vi "UHR-Fleezers Control (host) - 12.6.vi"() -> ()   [LabVIEW 2012] (continued)
        n1396 = property on="Green Laser ON" class="Bool (strict)"("Val(Sgnl)"="Green Laser ON/OFF") -> ()  [unwired: 2 in, 2 out]
      }
      event "Laser interlacing mode", "Green Laser ON", "Red Laser ON", "Blue Laser ON": Value Change {
        n1397 = event-data() -> ()  [unwired: 7 out]
        n1398 = local write "Green Laser ON/OFF"("Green Laser ON") -> ()
        n1399 = local write "Blue Laser ON/OFF"("Blue Laser ON") -> ()
        n1400 = local write "Red Laser ON/OFF"("Red Laser ON") -> ()
        n1401 = case shown="True" "Green Laser ON" {
          tunnel: "Laser interlacing mode" -> [_ w2024]
          tunnel: [enum32{"Laser ON", "Laser OFF", "Interlace"}."Laser OFF" ("Green laser mode") w2024] -> w2000
          tunnel: [FALSE w2020] -> w1999
          frame False {
          }
          frame True {
            n1402 = local read "Green FB On/Off"() -> (w2021:bool)
            n1403 = Equal?(x=w2024, y=enum32{"Laser ON", "Laser OFF", "Interlace"}."Interlace") -> (x = y?=w2022:bool)
            n1404 = And(x=w2022, y=w2021) -> (x .and. y?=w2020:bool)
          }
        }
        n1405 = case shown="True" "Red Laser ON" {
          tunnel: "Laser interlacing mode" -> [_ w2017]
          tunnel: [enum32{"Laser ON", "Laser OFF", "Interlace"}."Laser OFF" ("Green laser mode") w2017] -> w1996
          tunnel: [FALSE w2013] -> w1995
          frame False {
          }
          frame True {
            n1406 = local read "Red FB On/Off"() -> (w2014:bool)
            n1407 = Equal?(x=w2017, y=enum32{"Laser ON", "Laser OFF", "Interlace"}."Interlace") -> (x = y?=w2015:bool)
            n1408 = And(x=w2015, y=w2014) -> (x .and. y?=w2013:bool)
          }
        }
        n1409 = case shown="True" "Blue Laser ON" {
          tunnel: "Laser interlacing mode" -> [_ w2008]
          tunnel: [enum32{"Laser ON", "Laser OFF", "Interlace"}."Laser OFF" ("Green laser mode") w2008] -> w1992
          tunnel: [FALSE w2006] -> w1991
          frame False {
          }
          frame True {
            n1410 = local read "Blue FB On/Off"() -> (w2007:bool)
            n1411 = Equal?(x=w2008, y=enum32{"Laser ON", "Laser OFF", "Interlace"}."Interlace") -> (x = y?=w2009:bool)
            n1412 = And(x=w2009, y=w2007) -> (x .and. y?=w2006:bool)
          }
        }
        n1413 = xnode "Read/Write Control"("FPGA VI Reference In"=w2003, "error in"=w2001, "Operating Mode"=w2000, "Operating Mode 2"=w2000, "Green FB On/Off"=w1999, "Red Laser Operating Mode"=w1996, "RI Operating Mode 2"=w1996, "Red FB On/Off"=w1995, "BI Operating Mode (AO)"=w1992, "Blue Laser Operating Mode (D)"=w1992, "Blue FB On/Off"=w1991) -> ("error out"=w2002:errorcluster)  [unwired: 1 out]
      }
      event "Invert laser interlacing": Value Change {
        n1414 = event-data() -> ()  [unwired: 7 out]
        n1415 = xnode "Read/Write Control"("FPGA VI Reference In"=w2028, "error in"=w2026, "Invert GI"="Invert laser interlacing", "Invert GI 2"="Invert laser interlacing", "Invert RI"="Invert laser interlacing", "Invert RI 2"="Invert laser interlacing", "Invert BI (AO)"="Invert laser interlacing", "Invert BI (D)"="Invert laser interlacing") -> ("error out"=w2027:errorcluster)  [unwired: 1 out]
      }
      event "Green FB Setpoint (mV)", "Green FB Gains", "Green FB On/Off", "Green Intensity % (FB OFF)", "Green int current ON count adj": Value Change {
        n1416 = event-data() -> ()  [unwired: 7 out]
        n1417 = local read "Green FB Setpoint (mV)"() -> (w2039:dbl)
        n1418 = Multiply(x=w2039, y=3.2767) -> (x*y=w2038:dbl)
        n1419 = local read "Green Intensity % (FB OFF)"() -> (w2042:dbl)
        n1420 = Multiply(x=w2042, y=655.35) -> (x*y=w2043:dbl)
        n1421 = To Unsigned Word Integer(number=w2043) -> (unsigned 16bit integer=w2041:u16)
        n1422 = local read "Green int current ON count adj"() -> (w2045:u32)
        n1423 = local read "Laser interlacing mode"() -> (w2035:enum32{"Laser ON", "Laser OFF", "Interlace"})
        n1424 = local read "Green FB Gains"() -> (w2032:T9)
        n1425 = local read "Green Laser ON"() -> (w2036:bool)
        n1426 = local read "Green FB On/Off"() -> (w2046:bool)
        n1427 = Equal?(x=w2035, y=enum32{"Laser ON", "Laser OFF", "Interlace"}."Interlace") -> (x = y?=w2033:bool)
        n1428 = Unbundle By Name(w2032) -> ("proportional gain (Kc)"=w2031:i16, "integral gain (Kc*Ts/Ti)"=w2030:i16, "derivative gain (Kc*Td/Ts)"=w2029:i16)
        n1429 = Compound Arithmetic op=AND(w2033, w2046, w2036) -> (w2037:bool)
        n1430 = xnode "Read/Write Control"("FPGA VI Reference In"=w2049, "error in"=w2048, "Green FB Setpoint"=w2038, "Green FB On/Off"=w2037, "Current Out"=w2041, "Green int current ON count adj"=w2045, "P3"=w2031, "I3"=w2030, "D3"=w2029) -> ("error out"=w2047:errorcluster)  [unwired: 1 out]
      }
      event "Blue FB Setpoint (mV)", "Blue FB Gains", "Blue FB On/Off", "Blue Intensity % (FB OFF)", "Blue int AO ON count adjust": Value Change {
        # "16 bit analog out"
        n1431 = event-data() -> ()  [unwired: 7 out]
        n1432 = Multiply(x="Blue FB Setpoint (mV)", y=3.2767) -> (x*y=w2063:dbl)
        n1433 = Multiply(x="Blue Intensity % (FB OFF)", y=655.35) -> (x*y=w2066:dbl)
        n1434 = To Unsigned Word Integer(number=w2066) -> (unsigned 16bit integer=w2065:u16)
        n1435 = local read "Laser interlacing mode"() -> (w2061:enum32{"Laser ON", "Laser OFF", "Interlace"})
        n1436 = Unbundle By Name("Blue FB Gains") -> ("proportional gain (Kc)"=w2058:i16, "integral gain (Kc*Ts/Ti)"=w2057:i16, "derivative gain (Kc*Td/Ts)"=w2056:i16)
        n1437 = local read "Blue Laser ON"() -> (w2050:bool)
        n1438 = Equal?(x=w2061, y=enum32{"Laser ON", "Laser OFF", "Interlace"}."Interlace") -> (x = y?=w2059:bool)
        n1439 = Compound Arithmetic op=AND(w2059, "Blue FB On/Off", w2050) -> (w2062:bool)
        n1440 = xnode "Read/Write Control"("FPGA VI Reference In"=w2070, "error in"=w2069, "Blue FB Setpoint"=w2063, "Blue FB On/Off"=w2062, "BI Current Out"=w2065, "Blue current ON count adj (AO)"="Blue int AO ON count adjust", "P5"=w2058, "I5"=w2057, "D5"=w2056) -> ("error out"=w2068:errorcluster)  [unwired: 1 out]
      }
      event "Red FB Setpoint (mV)", "Red FB Gains", "Red FB On/Off", "Red Intensity % (FB OFF)": Value Change {
        n1441 = event-data() -> ()  [unwired: 7 out]
        n1442 = local read "Red FB Setpoint (mV)"() -> (w2082:dbl)
        n1443 = Multiply(x=w2082, y=3.2767) -> (x*y=w2081:dbl)
        n1444 = local read "Red Intensity % (FB OFF)"() -> (w2071:dbl)
        n1445 = Multiply(x=w2071, y=655.35) -> (x*y=w2085:dbl)
        n1446 = To Unsigned Word Integer(number=w2085) -> (unsigned 16bit integer=w2084:u16)
        n1447 = local read "Laser interlacing mode"() -> (w2078:enum32{"Laser ON", "Laser OFF", "Interlace"})
        n1448 = local read "Red FB Gains"() -> (w2075:T9)
        n1449 = local read "Red Laser ON"() -> (w2079:bool)
        n1450 = local read "Red FB On/Off"() -> (w2087:bool)
        n1451 = Equal?(x=w2078, y=enum32{"Laser ON", "Laser OFF", "Interlace"}."Interlace") -> (x = y?=w2076:bool)
        n1452 = Unbundle By Name(w2075) -> ("proportional gain (Kc)"=w2074:i16, "integral gain (Kc*Ts/Ti)"=w2073:i16, "derivative gain (Kc*Td/Ts)"=w2072:i16)
        n1453 = Compound Arithmetic op=AND(w2076, w2087, w2079) -> (w2080:bool)
        n1454 = xnode "Read/Write Control"("FPGA VI Reference In"=w2090, "error in"=w2089, "Red FB Setpoint"=w2081, "Red FB On/Off"=w2080, "RI Current Out"=w2084, "P4"=w2074, "I4"=w2073, "D4"=w2072) -> ("error out"=w2088:errorcluster)  [unwired: 1 out]
      }
      event "+ phase (APD 1 Gate)", "- phase (APD 1 Gate)", "+ phase (APD 2 Gate)", "- phase (APD 2 Gate)", "+ phase (APD 3 Gate)", "- phase (APD 3 Gate)", "+ phase (APD Acq)", "- phase (APD Acq)": Value Change {
        n1455 = event-data() -> ()  [unwired: 7 out]
        n1456 = local read "Phase Adj. (APD 1 Gate)"() -> (w2110:i16)
        n1457 = Or(x="- phase (APD 1 Gate)", y="+ phase (APD 1 Gate)") -> (x .or. y?=w2112:bool)
        n1458 = Negate(x=w2110) -> (-x=w2117:i16)
        n1459 = Select(t=w2117, s="+ phase (APD 1 Gate)", f=w2110) -> (s? t:f=w2116:i16)
        n1460 = local read "Phase Adj. (APD 2 Gate)"() -> (w2107:i16)
        n1461 = Or(x="- phase (APD 2 Gate)", y="+ phase (APD 2 Gate)") -> (x .or. y?=w2105:bool)
        n1462 = Negate(x=w2107) -> (-x=w2109:i16)
        n1463 = Select(t=w2109, s="+ phase (APD 2 Gate)", f=w2107) -> (s? t:f=w2106:i16)
        n1464 = Negate(x="Phase Adj. (APD 3 Gate)") -> (-x=w2104:i16)
        n1465 = Or(x="- phase (APD 3 Gate)", y="+ phase (APD 3 Gate)") -> (x .or. y?=w2100:bool)
        n1466 = Select(t=w2104, s="+ phase (APD 3 Gate)", f="Phase Adj. (APD 3 Gate)") -> (s? t:f=w2101:i16)
        n1467 = local read "Phase Adj. (APD Acq)"() -> (w2098:i16)
        n1468 = Or(x="- phase (APD Acq)", y="+ phase (APD Acq)") -> (x .or. y?=w2096:bool)
        n1469 = Negate(x=w2098) -> (-x=w2099:i16)
        n1470 = Select(t=w2099, s="+ phase (APD Acq)", f=w2098) -> (s? t:f=w2097:i16)
        n1471 = xnode "Read/Write Control"("FPGA VI Reference In"=w2119, "error in"=w2118, "Phase count adjustment (APD 1 Gate)"=w2116, "Phase count adjustment (APD 2 Gate)"=w2106, "Phase count adjustment (APD 3 Gate)"=w2101, "Phase Count Adjustment (APD Acq)"=w2097) -> ("FPGA VI Reference Out"=w2114:T20, "error out"=w2115:errorcluster)
        n1472 = xnode "Read/Write Control"("FPGA VI Reference In"=w2114, "error in"=w2115, "+ phase (APD 1 Gate)"=w2112, "+ phase (APD 2 Gate)"=w2105, "+ phase (APD 3 Gate)"=w2100, "+ phase (APD Acq)"=w2096) -> ("error out"=w2113:errorcluster)  [unwired: 1 out]
      }
      event "Invert APD Gate", "APD Gate ON Count", "APD Gate OFF Count", "APD Gate", "APD Integration Time (s)", "APD AO Scale Factor", "Duty Frequency (ON 1/N cycles)", "Interlace ON count", "Interlace OFF count": Value Change {
        n1473 = event-data() -> ()  [unwired: 7 out]
        n1474 = Add(x="Interlace ON count", y="Interlace OFF count") -> (x+y=w2125:u16)
        n1475 = Add(x="APD Gate ON Count", y="APD Gate OFF Count") -> (x+y=w2136:u16)
        n1476 = Multiply(x="Duty Frequency (ON 1/N cycles)", y=w2125) -> (x*y=w2121:u16)
        "Green AI Count" <- w2121
        "Red AI Count" <- w2121
        "Blue AI Count" <- w2121
        n1477 = Subtract(x=w2121, y="Interlace ON count") -> (x-y=w2124:u16)
        n1478 = Multiply(x=w2136, y="Duty Frequency (ON 1/N cycles)") -> (x*y=w2135:u16)
        n1479 = Subtract(x=w2135, y="APD Gate ON Count") -> (x-y=w2134:u16)
        n1480 = local read "DMA Update Period (s)"() -> (w2137:dbl)
        n1481 = Multiply(x="APD Integration Time (s)", y=40000000.0) -> (x*y=w2141:dbl)
        n1482 = Reciprocal(x="APD Integration Time (s)") -> (1/x=→"APD Acq Rate (Hz)":dbl)
        n1483 = To Unsigned Long Integer(number=w2141) -> (unsigned 32bit integer=w2127:u32)
        "APD Int. Count" <- w2127
        n1484 = local read "Number of APDs"() -> (w2120:u8)
        n1485 = Divide(x=w2137, y="APD Integration Time (s)") -> (x/y=w2139:dbl)
        n1486 = Multiply(x=w2120, y=w2139) -> (x*y=w2138:dbl)
        n1487 = local write "APD Samples/FIFO Acq."(w2139) -> ()
        n1488 = local write "APD Elements/DMA read"(w2138) -> ()
        n1489 = xnode "Read/Write Control"("FPGA VI Reference In"=w2145, "error in"=w2144, "Invert APD Gate"="Invert APD Gate", "APD Gate ON Count"="APD Gate ON Count", "APD Gate OFF Count"=w2134, "APD Acq Rate Count"=w2127, "APD Gate Operating Mode"="APD Gate", "APD AO scale factor"="APD AO Scale Factor", "Green interlace ON count"="Interlace ON count", "Green interlace OFF count"=w2124, "Green interlace ON count 2"="Interlace ON count", "Green interlace OFF count 2"=w2124, "Green FB Count"=w2121, "Red interlace ON count"="Interlace ON count", "Red interlace OFF count"="Interlace OFF count", "Blue ON count (AO)"="Interlace ON count", "Blue OFF count (AO)"="Interlace OFF count", "Blue interlace OFF count (D)"="Interlace OFF count", "Blue interlace ON count (D)"="Interlace ON count") -> ("error out"=w2143:errorcluster)  [unwired: 1 out]
      }
      event "Neg. TTrig FPGA": Value Change {
        n1490 = event-data() -> ()  [unwired: 7 out]
        n1491 = xnode "Read/Write Control"("FPGA VI Reference In"=w2148, "error in"=w2147, "TTrig Negate Pos"="Neg. TTrig FPGA") -> ()  [unwired: 2 out]
      }
      event "Test ttrig": Value Change {
        n1492 = event-data() -> ()  [unwired: 7 out]
        n1493 = xnode "Read/Write Control"("FPGA VI Reference In"=w2152, "error in"=w2151, "TTrig?"=TRUE) -> ("error out"=w2150:errorcluster)  [unwired: 1 out]
      }
      event "Number of F/B Scans (AOD)", "Scan Speed (nm/s)", "Scan BD", "Initial delta (MHz)", "Step Size (nm)", "Scan Range (nm)": Value Change {
        w2215 = 123.0  # AOM cal (nm/MHz)
        n1494 = event-data() -> ()  [unwired: 7 out]
        n1495 = local read "BD 1 Frequency 1 (MHz)"() -> (w2198:dbl)
        n1496 = local read "AOM X Cal (nm/MHz)"() -> (w2190:dbl)
        n1497 = local read "X RF Frequency Limits (MHz)"() -> (w2202:T16)
        n1498 = local read "Y RF Frequency Limits (MHz)"() -> (w2199:T16)
        n1499 = local read "BD 2 Frequency 1 (MHz)"() -> (w2204:dbl)
        n1500 = Negate(x="Scan Range (nm)") -> (-x=w2168:dbl)
        n1501 = Divide(x=w2168, y=w2190) -> (x/y=w2172:dbl)
        n1502 = Select(t=w2202, s="Scan BD", f=w2199) -> (s? t:f=w2201:T16)
        n1503 = Select(t=w2198, s="Scan BD", f=w2204) -> (s? t:f=w2203:dbl)
        n1504 = Unbundle By Name(w2201) -> ("Maximum"=w2210:dbl, "Minimum"=w2209:dbl)
        n1505 = Add(x=w2172, y=w2203) -> (x+y=w2207:dbl)
        n1506 = Divide(x=w2168, y="Step Size (nm)") -> (x/y=w2187:dbl)
        n1507 = Divide(x="Step Size (nm)", y=w2190) -> (x/y=w2196:dbl)
        n1508 = Absolute Value(x=w2187) -> (abs(x)=w2171:dbl)
        n1509 = Sign(1:w2168) -> (0:w2169:dbl)
        n1510 = In Range and Coerce(upper limit=w2210, x=w2207, lower limit=w2209) -> (coerced(x)=w2206:dbl, In Range?=w2208:bool)
        n1511 = To Unsigned Quad Integer(1:w2171) -> (0:w2186:u64)
        "Scan steps (AOD)" <- w2186
        n1512 = call "IR AOM freq to word.vi"("Frequency In (MHz)"=w2196) -> ("Frequency Word Out (double)"=w2193:dbl)
        n1513 = Multiply(x=w2169, y=w2193) -> (x*y=w2170:dbl)
        n1514 = Subtract(x=w2207, y=w2206) -> (x-y=w2205:dbl)
        n1515 = To Quad Integer(1:w2170) -> (0:w2192:i64)
        "Incr. int (AOD)" <- w2192
        n1516 = Subtract(x=w2172, y=w2205) -> (x-y=w2191:dbl)
        "Scan Range (MHz)" <- w2191
        n1517 = Select(t=w2172, s=w2208, f=w2191) -> (s? t:f=w2211:dbl)
        n1518 = Multiply(x=w2191, y=w2190) -> (x*y=w2189:dbl)
        n1519 = Decrement(x=w2186) -> (x-1=w2239:u64)
        n1520 = Negate(x=w2189) -> (-x=w2185:dbl)
        n1521 = local write "Scan Range (nm)"(w2185) -> ()
        n1522 = Divide(x=w2211, y=w2239) -> (x/y=w2195:dbl)
        "Scan Increment (MHz)" <- w2195
        n1523 = call "IR AOM freq to word.vi"("Frequency In (MHz)"=w2195) -> ("Frequency Word Out (double)"=w2194:dbl)
        n1524 = Divide(x="Step Size (nm)", y="Scan Speed (nm/s)") -> (x/y=w2182:dbl)
        n1525 = To Quad Integer(1:w2194) -> ()  [unwired: 1 out]
        n1526 = local read "Number Interlace Sets"() -> (w2166:u8)
        n1527 = local read "AI Count (ticks)"() -> (w2167:u16)
        n1528 = local read "Total Counts (ticks)"() -> (w2165:u16)
        n1529 = local read "# Samples/trap"() -> (w2197:u32)
        n1530 = Multiply(x=w2167, y=w2166) -> (x*y=w2164:u16)
        n1531 = Divide(x=w2165, y=w2164) -> (x/y=w2163:dbl)
        n1532 = Select(t=w2198, s="Scan BD", f=w2204) -> (s? t:f=w2236:dbl)
        "Initial freq. (MHz)" <- w2236
        n1533 = Add(x=w2211, y=w2236) -> (x+y=→"Final freq. (MHz)":dbl)
        n1534 = Divide(x=w2165, y=40000000.0) -> (x/y=w2181:dbl)
        n1535 = Divide(x=w2182, y=w2181) -> (x/y=w2180:dbl)
        n1536 = To Unsigned Quad Integer(1:w2180) -> (0:w2155:u64)
        n1537 = Quotient & Remainder(x=w2155, y=u64 2) -> (x-y*floor(x/y)=w2159:u64)  [unwired: 1 out]
        n1538 = Equal?(x=w2159, y=u64 0) -> (x = y?=w2157:bool)
        n1539 = Decrement(x=w2155) -> (x-1=w2156:u64)
        n1540 = Select(t=w2155, s=w2157, f=w2156) -> (s? t:f=w2154:u64)
        "Cycles/step (AOD)" <- w2154
        n1541 = xnode "Read/Write Control"("FPGA VI Reference In"=w2247, "error in"=w2246, "Scan steps"=w2186, "Number of scans"="Number of F/B Scans (AOD)", "Cycles per step"=w2154, "Scan freq.  increment"=w2192, "Scan BD"="Scan BD") -> ("error out"=w2245:errorcluster)  [unwired: 1 out]
        n1542 = Multiply(x=w2186, y=w2154) -> (x*y=w2240:u64)
        n1543 = Multiply(x=w2240, y=u64 2) -> (x*y=w2162:u64)
        n1544 = Multiply(x=w2163, y=w2162) -> (x*y=w2161:dbl)
        "Data points/scan (f/b)" <- w2161
        n1545 = Multiply(x=w2161, y="Number of F/B Scans (AOD)") -> (x*y=w2243:dbl)
        "Data points/scans" <- w2243
        n1546 = Divide(x=w2243, y=w2197) -> (x/y=→"N sets should be saved":dbl)
        n1547 = Multiply(x=w2240, y=w2181) -> (x*y=w2179:dbl)
        "Time/Scan (s) (AOD)" <- w2179
        n1548 = Select(t=w2211, s="Scan BD", f=0.0) -> (s? t:f=w2237:dbl)
        n1549 = Select(t=0.0, s="Scan BD", f=w2211) -> (s? t:f=w2233:dbl)
        n1550 = local read "BD 2 Frequency 2 (MHz)"() -> (w2229:dbl)
        n1551 = local read "BD 1 Frequency 2 (MHz)"() -> (w2232:dbl)
        n1552 = Add(x=w2233, y=w2204) -> (x+y=w2230:dbl)
        n1553 = Add(x=w2198, y=w2237) -> (x+y=w2231:dbl)
        n1554 = Multiply(x=w2179, y=2.0) -> (x*y=w2178:dbl)
        n1555 = Multiply(x=w2178, y="Number of F/B Scans (AOD)") -> (x*y=w2175:dbl)
        n1556 = Divide(x=w2175, y=60.0) -> (x/y=→"Time to Finish All (min)":dbl)
        n1557 = Add(x="Trap 2 Bead Size (nm)", y="Trap 1 Bead Size (nm)") -> (x+y=w2219:dbl)
        n1558 = Divide(x=w2219, y=2.0) -> (x/y=w2213:dbl)
        n1559 = local read "Initial delta (MHz)"() -> (w2216:dbl)
        n1560 = Subtract(x=w2230, y=w2229) -> (x-y=w2227:dbl)
        n1561 = Subtract(x=w2231, y=w2232) -> (x-y=w2228:dbl)
        n1562 = Square(x=w2227) -> (x^2=w2226:dbl)
        n1563 = Square(x=w2228) -> (x^2=w2225:dbl)
        n1564 = Add(x=w2225, y=w2226) -> (x+y=w2224:dbl)
        n1565 = Square Root(x=w2224) -> (sqrt(x)=w2223:dbl)
        "Final delta (MHz)" <- w2223
        n1566 = Multiply(x=w2215, y=w2223) -> (x*y=w2222:dbl)
        n1567 = Multiply(x=w2216, y=w2215) -> (x*y=w2214:dbl)
        n1568 = Subtract(x=w2214, y=w2213) -> (x-y=→"Initial sep (nm)":dbl)
        n1569 = Subtract(x=w2222, y=w2213) -> (x-y=→"Final sep (nm)":dbl)
      }
      event "Freq or Amp switch first", "Swap F1 and F2", "Freq switch delay", "Amp switch delay": Value Change {
        n1570 = event-data() -> ()  [unwired: 7 out]
        n1571 = local read "Amp switch delay"() -> (w2248:u16)
        n1572 = local read "Swap F1 and F2"() -> (w2249:bool)
        n1573 = xnode "Read/Write Control"("FPGA VI Reference In"=w2252, "error in"=w2251, "Swap F1 and F2"=w2249, "Amp switch delay"=w2248) -> ("error out"=w2250:errorcluster)  [unwired: 1 out]
      }
      event "Scan steps (MCL)", "Number of scans (MCL)", "Scan Range (V)\n(of steps)", "2D or 1D Scan", "N APD Samp/step", "Fast Scan Dir", "Continuous MCL Scanning", "Scan lines (y)": Value Change {
        w2254 = 32767.0 ("y")
        n1574 = event-data() -> ()  [unwired: 7 out]
        n1575 = Select(t="Scan lines (y)", s="2D or 1D Scan", f="Number of scans (MCL)") -> (s? t:f=w2259:u64)
        n1576 = Decrement(x="Scan steps (MCL)") -> (x-1=w2275:u64)
        n1577 = Divide(x="Scan Range (V)\n(of steps)", y=w2275) -> (x/y=w2274:dbl)
        "Desired Scan Incr (V)" <- w2274
        n1578 = local read "APD Integration Time (s)"() -> (w2267:dbl)
        n1579 = Multiply(x=w2274, y=w2254) -> (x*y=w2283:dbl)
        n1580 = Divide(x=w2283, y=10.0) -> (x/y=w2273:dbl)
        "Desired incr (int)" <- w2273
        n1581 = local read "Update Count (MCL)"() -> (w2279:u32)
        n1582 = Round Toward -Infinity(1:w2273) -> (0:w2282:dbl)
        n1583 = To Word Integer(number=w2282) -> (16bit integer=w2257:i16)
        "Actual Incr. int (MCL)" <- w2257
        n1584 = Multiply(x=w2267, y=40000000.0) -> (x*y=w2280:dbl)
        n1585 = Divide(x=w2280, y=w2279) -> (x/y=w2278:dbl)
        n1586 = Multiply(x=i16 10, y=w2257) -> (x*y=w2255:i16)
        n1587 = Multiply(x="N APD Samp/step", y=w2278) -> (x*y=w2277:dbl)
        "Cycles/step (MCL)" <- w2277
        n1588 = Divide(x=w2255, y=w2254) -> (x/y=→"Actual MCL Inc (V)":dbl)
        n1589 = Multiply(x="N APD Samp/step", y="Scan steps (MCL)") -> (x*y=w2269:dbl)
        n1590 = local read "APD Samples/FIFO Acq."() -> (w2266:dbl)
        n1591 = Multiply(x=w2269, y=u64 2) -> (x*y=w2268:dbl)
        "Data points/scan (f+b)" <- w2268
        n1592 = Multiply(x=w2268, y=w2259) -> (x*y=w2286:dbl)
        "Data points/scans (MCL)" <- w2286
        n1593 = Multiply(x=w2267, y=w2268) -> (x*y=w2260:dbl)
        "Time/f+b scan (s) (MCL)" <- w2260
        n1594 = Divide(x=w2286, y=w2266) -> (x/y=→"N sets should be saved (MCL)":dbl)
        n1595 = Multiply(x=w2260, y=w2259) -> (x*y=→"Total Time (s)":dbl)
        n1596 = Not(x="Fast Scan Dir") -> (.not. x?=w2264:bool)
        n1597 = xnode "Read/Write Control"("FPGA VI Reference In"=w2290, "error in"=w2289, "Scan steps (MCL)"="Scan steps (MCL)", "Number of scans (MCL)"=w2259, "Cycles per step (MCL)"=w2277, "Scan freq.  increment (MCL)"=w2257, "1D or 2D Scan?"="2D or 1D Scan", "MCL Scan Axis"=w2264, "Cont. Scan (MCL)"="Continuous MCL Scanning") -> ("error out"=w2288:errorcluster)  [unwired: 1 out]
      }
      event "Read Cal": Value Change {
        w2292 = 1000.0 ("y")
        n1598 = event-data() -> ()  [unwired: 7 out]
        n1599 = local read "Save file name"() -> (w2317:path)
        n1600 = local write "Read Cal"(FALSE ("Read Cal")) -> ()
        n1601 = Strip Path(path=w2317) -> (stripped path=w2316:path)  [unwired: 1 out]
        n1602 = Path To String(path=w2316) -> (string=w2315:string)
        n1603 = Concatenate Strings(w2315, "\\current.cal" ("string")) -> (w2313:string)
        n1604 = String To Path(string=w2313) -> (path=w2312:path)
        n1605 = Open/Create/Replace File(file path (use dialog)=w2312, operation (0:open)=T29."open", access (0:read/write)=enum16{"read/write", "read-only", "write-only"}."read-only") -> (refnum out=w2320:refnum<file>, error out=w2306:errorcluster)  [unwired: 1 in, 3 out]
        n1606 = Deny Access(4:w2306, 7:w2320) -> (0:w2305:errorcluster, 3:w2311:refnum<file>)  [unwired: 1 out]
        n1607 = Read from Binary File(5:0.0, 8:w2305, 9:T28."big-endian, network order" ("byte order (0:big-endian, network order)"), 10:-1 ("count (1)"), 11:w2311) -> (0:w2304:errorcluster, 2:w2302:dbl[], 3:w2307:refnum<file>)  [unwired: 2 out]
        n1608 = Array To Cluster(array=w2302) -> (cluster=w2301:T31)
        n1609 = Unbundle(w2301) -> ("[0]"=w2300:dbl, "[1]"=w2299:dbl, "[2]"=w2298:dbl, "[3]"=w2297:dbl, "[4]"=w2296:dbl, "[5]"=w2295:dbl)
        n1610 = Close File(refnum=w2307, error in=w2304) -> (error out=→"Read cal error":errorcluster)  [unwired: 1 out]
        n1611 = Multiply(x=w2295, y=w2292) -> (x*y=w2293:dbl)
        n1612 = local write "T2 kappa_x (pN/nm)"(w2297) -> ()
        n1613 = local write "T1 kappa_x (pN/nm)"(w2298) -> ()
        n1614 = local write "T1 alpha_x (nm/V)"(w2300) -> ()
        n1615 = local write "T2 alpha_x (nm/V)"(w2299) -> ()
        n1616 = Multiply(x=w2296, y=w2292) -> (x*y=w2294:dbl)
        n1617 = local write "T1 offset_x (mV)"(w2294) -> ()
        n1618 = local write "T2 offset_x (mV)"(w2293) -> ()
      }
      event "Abort MCL Scan": Value Change {
        n1619 = event-data() -> ()  [unwired: 7 out]
        n1620 = local write "MCL Scanning"(FALSE ("MCL Scanning")) -> ()
        n1621 = xnode "Read/Write Control"("FPGA VI Reference In"=w2325, "error in"=w2324, "Abort scan (MCL)"="Abort MCL Scan") -> ("error out"=w2323:errorcluster)  [unwired: 1 out]
      }
      event "Update Count (MCL)": Value Change {
        n1622 = event-data() -> ()  [unwired: 7 out]
        n1623 = xnode "Read/Write Control"("FPGA VI Reference In"=w2329, "error in"=w2328, "MCL count"="Update Count (MCL)") -> ("error out"=w2327:errorcluster)  [unwired: 1 out]
      }
      event "+ phase (MCL)", "- phase (MCL)": Value Change {
        n1624 = event-data() -> ()  [unwired: 7 out]
        n1625 = Or(x="- phase (MCL)", y="+ phase (MCL)") -> (x .or. y?=w2332:bool)
        n1626 = Negate(x="Phase adjust (MCL)") -> (-x=w2338:i16)
        n1627 = Select(t=w2338, s="+ phase (MCL)", f="Phase adjust (MCL)") -> (s? t:f=w2336:i16)
        n1628 = xnode "Read/Write Control"("FPGA VI Reference In"=w2340, "error in"=w2339, "Phase count adjustment (MCL)"=w2336) -> ("FPGA VI Reference Out"=w2333:T20, "error out"=w2334:errorcluster)
        n1629 = xnode "Read/Write Control"("FPGA VI Reference In"=w2333, "error in"=w2334, "+ phase (MCL)"=w2332) -> ("error out"=w2331:errorcluster)  [unwired: 1 out]
      }
      event "Abort AOD Scan": Value Change {
        n1630 = event-data() -> ()  [unwired: 7 out]
        n1631 = xnode "Read/Write Control"("FPGA VI Reference In"=w2344, "error in"=w2343, "Abort scan"="Abort AOD Scan") -> ("error out"=w2342:errorcluster)  [unwired: 1 out]
      }
      event "Continuous AOD Scanning": Value Change {
        n1632 = event-data() -> ()  [unwired: 7 out]
        n1633 = xnode "Read/Write Control"("FPGA VI Reference In"=w2348, "error in"=w2347, "Cont. Scan"="Continuous AOD Scanning") -> ("error out"=w2346:errorcluster)  [unwired: 1 out]
      }
      event "Index": Value Change {
        n1634 = event-data() -> ()  [unwired: 7 out]
        n1635 = call "Create new save file.vi"("Insert"="", "Ext"=".dat" ("string"), "Index In"="Index") -> ("Path Out"=→"Save file name":path, "Index Out"=w2349:dbl)
        "Save index" <- w2349
        n1636 = local write "Index"(w2349) -> ()
      }
      event "AO1", "AO2": Value Change {
        w2364 = 10.0 ("y")
        w2363 = 32767.0 ("y")
        n1637 = event-data() -> ()  [unwired: 7 out]
        n1638 = local read "AO2"() -> (w2362:dbl)
        n1639 = local read "AO1"() -> (w2359:dbl)
        n1640 = Multiply(x=w2359, y=w2363) -> (x*y=w2358:dbl)
        n1641 = Multiply(x=w2362, y=w2363) -> (x*y=w2361:dbl)
        n1642 = Divide(x=w2358, y=w2364) -> (x/y=w2357:dbl)
        n1643 = Divide(x=w2361, y=w2364) -> (x/y=w2360:dbl)
        n1644 = To Word Integer(number=w2357) -> (16bit integer=w2365:i16)
        n1645 = To Word Integer(number=w2360) -> (16bit integer=w2366:i16)
        n1646 = xnode "Read/Write Control"("FPGA VI Reference In"=w2356, "error in"=w2355, "AO1"=w2365, "AO2"=w2366) -> ("error out"=w2354:errorcluster)  [unwired: 1 out]
      }
      event "Inject Pump 1": Value Change {
        n1647 = event-data() -> ()  [unwired: 7 out]
        n1648 = local read "Use Harvard pumps\nfor beads (else Chemyx)"() -> (w2368:bool)
        n1649 = case shown="True" w2368 {
          tunnel: "Inject Pump 1" -> [w2372 w2410]
          tunnel: w2367 -> [_ w2411]
          frame False {
            n1650 = local read "Pump write delay (ms)"() -> (w2371:dbl)
            n1651 = local read "Chemyx Syringe Pump Serial Port"() -> (w2370:refnum<visa-resource-name>)
            n1652 = case shown="True" w2372 {
              tunnel: w2371 -> [w2378 w2392]
              tunnel: w2370 -> [w2375 w2391]
              frame False {
                n1653 = flat-sequence {
                  tunnel: w2375 -> [w2379]
                  tunnel: [w2379] -> w2376
                  tunnel: w2378 -> [_]
                  tunnel: [w2382] -> w2377
                  tunnel: w2376 -> [w2382]
                  tunnel: w2377 -> [w2383]
                  tunnel: [w2383] -> w2373
                  tunnel: [w2385] -> w2374
                  tunnel: w2373 -> [w2385]
                  tunnel: w2374 -> [w2387]
                  frame #0 {
                    n1654 = call "Write to pump.vi"("string"="enter pump1", "VISA resource name"=w2379) -> ()  [unwired: 1 out]
                  }
                  frame #1 {
                    n1655 = Wait (ms)(milliseconds to wait="Pump pause delay (ms)") -> ()  [unwired: 1 out]
                  }
                  frame #2 {
                    n1656 = call "Write to pump.vi"("string"="stop", "VISA resource name"=w2383) -> ()  [unwired: 1 out]
                  }
                  frame #3 {
                    n1657 = Wait (ms)(milliseconds to wait=u32 500) -> ()  [unwired: 1 out]
                  }
                  frame #4 {
                    n1658 = call "Write to pump.vi"("string"="stop", "VISA resource name"=w2387) -> ()  [unwired: 1 out]
                  }
                }
              }
              frame True {
                n1659 = flat-sequence {
                  tunnel: w2391 -> [w2401]
                  tunnel: w2392 -> [w2396]
                  tunnel: w2392 -> [w2403]
                  tunnel: w2391 -> [w2404]
                  tunnel: [w2404] -> w2389
                  tunnel: [w2406] -> w2390
                  tunnel: w2389 -> [w2406]
                  tunnel: w2390 -> [w2408]
                  frame #0 {
                    n1660 = local read "All Pump Parameters"() -> (w2395:T5)
                    n1661 = Unbundle By Name(w2395) -> ("Pump 1"=w2402:T32)
                    n1662 = call "Set pump parameters.vi"("Pump write delay (ms)"=w2396, "Volume (uL)"="Ch 1 Inject Volume (uL)", "Rate (uL/h)"="Ch 1 Inject Rate (ul/h)", "Units"=4.0, "Pump #"=1.0, "Pump Parameters In"=w2402, "VISA resource name"=w2401) -> ("Pump Parameters Out"=w2394:T32)  [unwired: 3 in]
                    n1663 = Bundle By Name(cluster=w2395, "Pump 1"=w2394) -> (w2393:T5)
                    n1664 = local write "All Pump Parameters"(w2393) -> ()
                  }
                  frame #1 {
                    n1665 = Wait (ms)(milliseconds to wait=w2403) -> ()  [unwired: 1 out]
                  }
                  frame #2 {
                    n1666 = call "Write to pump.vi"("string"="start", "VISA resource name"=w2404) -> ()  [unwired: 1 out]
                  }
                  frame #3 {
                    n1667 = Wait (ms)(milliseconds to wait=u32 500) -> ()  [unwired: 1 out]
                  }
                  frame #4 {
                    n1668 = call "Write to pump.vi"("string"="start", "VISA resource name"=w2408) -> ()  [unwired: 1 out]
                  }
                }
              }
            }
          }
          frame True {
            n1669 = case shown="False" w2410 {
              tunnel: w2411 -> [w2412 w2422]
              frame False {
                n1670 = flat-sequence {
                  tunnel: w2412 -> [w2414]
                  frame #0 {
                    n1671 = local write "Flushing P1"(FALSE ("Flushing P1")) -> ()
                    n1672 = Concatenate Strings("stop" ("string"), "\r") -> (w2416:string)
                    n1673 = VISA Write(VISA resource name=w2414, write buffer=w2416) -> ()  [unwired: 1 in, 3 out]
                  }
                  frame #1 {
                    n1674 = property on="Clear Volume P1" class="Bool (strict)"("Val(Sgnl)"=TRUE ("Value (Signaling)")) -> ()  [unwired: 2 in, 2 out]
                  }
                }
              }
              frame True {
                n1675 = local read "Normal Flow Rate (ul/h) P1"() -> (w2420:dbl)
                n1676 = Number To Decimal String(number=w2420) -> (decimal integer string=w2426:string)  [unwired: 1 in]
                n1677 = Concatenate Strings("irate  " ("string"), w2426, " u/h" ("string"), "\r") -> (w2424:string)
                n1678 = VISA Write(VISA resource name=w2422, write buffer=w2424) -> (VISA resource name out=w2421:refnum<visa-resource-name>)  [unwired: 1 in, 2 out]
                n1679 = Concatenate Strings("irun" ("string"), "\r") -> (w2428:string)
                n1680 = VISA Write(VISA resource name=w2421, write buffer=w2428) -> ()  [unwired: 1 in, 3 out]
              }
            }
          }
        }
      }
      event "Inject Pump 3": Value Change {
        n1681 = event-data() -> ()  [unwired: 7 out]
        n1682 = local read "Use Harvard pumps\nfor beads (else Chemyx)"() -> (w2431:bool)
        n1683 = case shown="True" w2431 {
          tunnel: "Inject Pump 3" -> [w2435 w2474]
          tunnel: w2430 -> [_ w2473]
          frame False {
            n1684 = local read "Pump write delay (ms)"() -> (w2434:dbl)
            n1685 = case shown="True" w2435 {
              tunnel: w2434 -> [w2441 w2455]
              tunnel: "Chemyx Syringe Pump Serial Port" -> [w2438 w2454]
              frame False {
                n1686 = flat-sequence {
                  tunnel: w2438 -> [w2442]
                  tunnel: [w2442] -> w2439
                  tunnel: w2441 -> [_]
                  tunnel: [w2445] -> w2440
                  tunnel: w2439 -> [w2445]
                  tunnel: w2440 -> [w2446]
                  tunnel: [w2446] -> w2436
                  tunnel: [w2448] -> w2437
                  tunnel: w2436 -> [w2448]
                  tunnel: w2437 -> [w2450]
                  frame #0 {
                    n1687 = call "Write to pump.vi"("string"="enter pump3", "VISA resource name"=w2442) -> ()  [unwired: 1 out]
                  }
                  frame #1 {
                    n1688 = local read "Pump pause delay (ms)"() -> (w2444:u32)
                    n1689 = Wait (ms)(milliseconds to wait=w2444) -> ()  [unwired: 1 out]
                  }
                  frame #2 {
                    n1690 = call "Write to pump.vi"("string"="stop", "VISA resource name"=w2446) -> ()  [unwired: 1 out]
                  }
                  frame #3 {
                    n1691 = Wait (ms)(milliseconds to wait=u32 0) -> ()  [unwired: 1 out]
                  }
                  frame #4 {
                    n1692 = call "Write to pump.vi"("string"="stop", "VISA resource name"=w2450) -> ()  [unwired: 1 out]
                  }
                }
              }
              frame True {
                n1693 = flat-sequence {
                  tunnel: w2454 -> [w2464]
                  tunnel: w2455 -> [w2459]
                  tunnel: w2455 -> [w2466]
                  tunnel: w2454 -> [w2467]
                  tunnel: [w2467] -> w2453
                  tunnel: [w2470] -> w2452
                  tunnel: w2453 -> [w2470]
                  tunnel: w2452 -> [w2471]
                  frame #0 {
                    n1694 = local read "All Pump Parameters"() -> (w2458:T5)
                    n1695 = Unbundle By Name(w2458) -> ("Pump 3"=w2465:T32)
                    n1696 = call "Set pump parameters.vi"("Pump write delay (ms)"=w2459, "Volume (uL)"="Ch 3 Inject Volume (uL)", "Rate (uL/h)"="Ch 3 Inject Rate (ul/h)", "Units"=4.0, "Pump #"=3.0, "Pump Parameters In"=w2465, "VISA resource name"=w2464) -> ("Pump Parameters Out"=w2457:T32)  [unwired: 3 in]
                    n1697 = Bundle By Name(cluster=w2458, "Pump 3"=w2457) -> (w2456:T5)
                    n1698 = local write "All Pump Parameters"(w2456) -> ()
                  }
                  frame #1 {
                    n1699 = Wait (ms)(milliseconds to wait=w2466) -> ()  [unwired: 1 out]
                  }
                  frame #2 {
                    n1700 = call "Write to pump.vi"("string"="start", "VISA resource name"=w2467) -> ()  [unwired: 1 out]
                  }
                  frame #3 {
                    n1701 = Wait (ms)(milliseconds to wait=u32 500) -> ()  [unwired: 1 out]
                  }
                  frame #4 {
                    n1702 = call "Write to pump.vi"("string"="start", "VISA resource name"=w2471) -> ()  [unwired: 1 out]
                  }
                }
              }
            }
          }
          frame True {
            n1703 = case shown="False" w2474 {
              tunnel: w2473 -> [w2475 w2482]
              frame False {
                n1704 = flat-sequence {
                  tunnel: w2475 -> [w2477]
                  frame #0 {
                    n1705 = local write "Flushing P3"(FALSE ("Flushing P3")) -> ()
                    n1706 = Concatenate Strings("stop" ("string"), "\r") -> (w2479:string)
                    n1707 = VISA Write(VISA resource name=w2477, write buffer=w2479) -> ()  [unwired: 1 in, 3 out]
                  }
                  frame #1 {
                    n1708 = property on="Clear Volume P3" class="Bool (strict)"("Val(Sgnl)"=TRUE ("Value (Signaling)")) -> ()  [unwired: 2 in, 2 out]
                  }
                }
              }
              frame True {
                n1709 = local read "Normal Flow Rate (ul/h) P3"() -> (w2483:dbl)
                n1710 = Number To Decimal String(number=w2483) -> (decimal integer string=w2489:string)  [unwired: 1 in]
                n1711 = Concatenate Strings("irate  " ("string"), w2489, " u/h" ("string"), "\r") -> (w2487:string)
                n1712 = VISA Write(VISA resource name=w2482, write buffer=w2487) -> (VISA resource name out=w2485:refnum<visa-resource-name>)  [unwired: 1 in, 2 out]
                n1713 = Concatenate Strings("irun" ("string"), "\r") -> (w2491:string)
                n1714 = VISA Write(VISA resource name=w2485, write buffer=w2491) -> ()  [unwired: 1 in, 3 out]
              }
            }
          }
        }
      }
      event "Inject Pump 2": Value Change {
        n1715 = event-data() -> ()  [unwired: 7 out]
        n1716 = local read "Pump write delay (ms)"() -> (w2495:dbl)
        n1717 = flat-sequence {
          tunnel: w2493 -> [w2508]
          tunnel: w2495 -> [w2504]
          tunnel: "Inject Pump 2" -> [_]
          tunnel: w2495 -> [w2510]
          tunnel: w2493 -> [w2511]
          frame #0 {
            n1718 = local read "All Pump Parameters"() -> (w2503:T5)
            n1719 = Multiply(x=60.0, y="Flush Center Ch Rate (ul/m)") -> (x*y=w2500:dbl)
            n1720 = Unbundle By Name(w2503) -> ("Pump 2"=w2509:T32)
            n1721 = call "Set pump parameters.vi"("Pump write delay (ms)"=w2504, "Volume (uL)"="Flush Center Ch Volume (uL)", "Rate (uL/h)"=w2500, "Units"=3.0, "Pump #"=2.0, "Pump Parameters In"=w2509, "VISA resource name"=w2508) -> ("Pump Parameters Out"=w2502:T32)  [unwired: 3 in]
            n1722 = Bundle By Name(cluster=w2503, "Pump 2"=w2502) -> (w2501:T5)
            n1723 = local write "All Pump Parameters"(w2501) -> ()
            n1724 = Add(x="Flush Center Ch Volume (uL)", y="Total Volume\nFlushed (uL)") -> (x+y=w2497:dbl)
            n1725 = local write "Total Volume\nFlushed (uL)"(w2497) -> ()
          }
          frame #1 {
            n1726 = Wait (ms)(milliseconds to wait=w2510) -> ()  [unwired: 1 out]
          }
          frame #2 {
            n1727 = call "Write to pump.vi"("string"="start", "VISA resource name"=w2511) -> ()  [unwired: 1 out]
          }
        }
        n1728 = local read "Chemyx Syringe Pump Serial Port"() -> (w2493:refnum<visa-resource-name>)
      }
      event "Sample Channel\nFlow": Value Change {
        n1729 = event-data() -> ()  [unwired: 7 out]
        n1730 = Select(t="irun" ("string"), s="Sample Channel\nFlow", f="stop" ("string")) -> (s? t:f=w2515:string)
        n1731 = Concatenate Strings(w2515, "\r") -> (w2518:string)
        n1732 = VISA Write(VISA resource name=w2513, write buffer=w2518) -> ()  [unwired: 1 in, 3 out]
      }
      event "Start Flow": Value Change {
        n1733 = event-data() -> ()  [unwired: 7 out]
        n1734 = local write "Sample Channel\nFlow"(TRUE ("Sample Channel\nFlow")) -> ()
        n1735 = local write "Start Flow"(FALSE ("Start Flow")) -> ()
        n1736 = Concatenate Strings("irun" ("string"), "\r") -> (w2524:string)
        n1737 = VISA Write(VISA resource name=w2520, write buffer=w2524) -> ()  [unwired: 1 in, 3 out]
      }
      event "Stop Flow": Value Change {
        w2526 = FALSE ("Stop Flow")
        n1738 = event-data() -> ()  [unwired: 7 out]
        n1739 = local write "Stop Flow"(w2526) -> ()
        n1740 = local write "Sample Channel\nFlow"(w2526) -> ()
        n1741 = Concatenate Strings("stop" ("string"), "\r") -> (w2529:string)
        n1742 = VISA Write(VISA resource name=w2527, write buffer=w2529) -> ()  [unwired: 1 in, 3 out]
      }
      event "Flow rate (uL/h)": Value Change {
        n1743 = event-data() -> ()  [unwired: 7 out]
        n1744 = Number To Decimal String(number="Flow rate (uL/h)") -> (decimal integer string=w2536:string)  [unwired: 1 in]
        n1745 = Concatenate Strings("irate  " ("string"), w2536, " u/h" ("string"), "\r") -> (w2535:string)
        n1746 = VISA Write(VISA resource name=w2532, write buffer=w2535) -> ()  [unwired: 1 in, 3 out]
      }
      event "Flush Sample": Value Change {
        n1747 = event-data() -> ()  [unwired: 7 out]
        n1748 = flat-sequence {
          tunnel: w2541 -> [w2569]
          tunnel: [w2549] -> w2540
          tunnel: [w2543] -> w2538
          tunnel: w2540 -> [w2573]
          tunnel: [w2573] -> w2539
          tunnel: w2538 -> [w2572]
          tunnel: w2539 -> [w2578]
          frame #0 {
            # "set paramaters (rate, volume) for flush, clear volume"
            n1749 = Number To Decimal String(number="Flush rate (uL/m)") -> (decimal integer string=w2565:string)  [unwired: 1 in]
            n1750 = Concatenate Strings("irate  " ("string"), w2565, " u/m" ("string"), "\r") -> (w2567:string)
            n1751 = VISA Write(VISA resource name=w2569, write buffer=w2567) -> (VISA resource name out=w2563:refnum<visa-resource-name>)  [unwired: 1 in, 2 out]
            n1752 = Reciprocal(x="Flush rate (uL/m)") -> (1/x=w2546:dbl)
            n1753 = Number To Decimal String(number="Volume (uL)") -> (decimal integer string=w2554:string)  [unwired: 1 in]
            n1754 = Multiply(x="Volume (uL)", y=w2546) -> (x*y=w2545:dbl)
            n1755 = Concatenate Strings("tvolume  " ("string"), w2554, " u" ("string"), "\r") -> (w2552:string)
            n1756 = Multiply(x=w2545, y=60000.0) -> (x*y=w2543:dbl)
            n1757 = VISA Write(VISA resource name=w2563, write buffer=w2552) -> (VISA resource name out=w2551:refnum<visa-resource-name>)  [unwired: 1 in, 2 out]
            n1758 = Concatenate Strings("cvolume" ("string"), "\r") -> (w2550:string)
            n1759 = VISA Write(VISA resource name=w2551, write buffer=w2550) -> (VISA resource name out=w2561:refnum<visa-resource-name>)  [unwired: 1 in, 2 out]
            n1760 = Concatenate Strings("irun" ("string"), "\r") -> (w2559:string)
            n1761 = VISA Write(VISA resource name=w2561, write buffer=w2559) -> (VISA resource name out=w2549:refnum<visa-resource-name>)  [unwired: 1 in, 2 out]
          }
          frame #1 {
            # "Have to wait until\nflow is done to reset\nrate"
            n1762 = Add(x=w2572, y=100.0) -> (x+y=w2571:dbl)
            n1763 = Wait (ms)(milliseconds to wait=w2571) -> ()  [unwired: 1 out]
          }
          frame #2 {
            # "reset flow rate to usual flow rate"
            n1764 = local read "Flow rate (uL/h)"() -> (w2584:dbl)
            n1765 = Number To Decimal String(number=w2584) -> (decimal integer string=w2582:string)  [unwired: 1 in]
            n1766 = Concatenate Strings("irate  " ("string"), w2582, " u/h" ("string"), "\r") -> (w2580:string)
            n1767 = VISA Write(VISA resource name=w2578, write buffer=w2580) -> (VISA resource name out=w2574:refnum<visa-resource-name>)  [unwired: 1 in, 2 out]
            n1768 = Concatenate Strings("cvolume" ("string"), "\r") -> (w2575:string)
            n1769 = VISA Write(VISA resource name=w2574, write buffer=w2575) -> ()  [unwired: 1 in, 3 out]
          }
        }
      }
      event "Flush Pump 3": Value Change {
        n1770 = event-data() -> ()  [unwired: 7 out]
        n1771 = flat-sequence {
          tunnel: w2585 -> [w2588]
          frame #0 {
            # "set paramaters (rate, volume) for flush, clear volume"
            n1772 = Number To Decimal String(number="Flush rate (uL/m) P3") -> (decimal integer string=w2610:string)  [unwired: 1 in]
            n1773 = local write "Inject Pump 3"(TRUE ("Inject Pump 3")) -> ()
            n1774 = Concatenate Strings("irate  " ("string"), w2610, " u/m" ("string"), "\r") -> (w2612:string)
            n1775 = VISA Write(VISA resource name=w2588, write buffer=w2612) -> (VISA resource name out=w2608:refnum<visa-resource-name>)  [unwired: 1 in, 2 out]
            n1776 = Reciprocal(x="Flush rate (uL/m) P3") -> (1/x=w2592:dbl)
            n1777 = Number To Decimal String(number="Volume (uL) P3") -> (decimal integer string=w2599:string)  [unwired: 1 in]
            n1778 = Multiply(x="Volume (uL) P3", y=w2592) -> (x*y=w2591:dbl)
            n1779 = Concatenate Strings("tvolume  " ("string"), w2599, " u" ("string"), "\r") -> (w2597:string)
            n1780 = Multiply(x=w2591, y=60.0) -> (x*y=→"HP3 Flush Time (s)":dbl)
            n1781 = VISA Write(VISA resource name=w2608, write buffer=w2597) -> (VISA resource name out=w2596:refnum<visa-resource-name>)  [unwired: 1 in, 2 out]
            n1782 = Concatenate Strings("cvolume" ("string"), "\r") -> (w2595:string)
            n1783 = VISA Write(VISA resource name=w2596, write buffer=w2595) -> (VISA resource name out=w2606:refnum<visa-resource-name>)  [unwired: 1 in, 2 out]
            n1784 = Concatenate Strings("irun" ("string"), "\r") -> (w2604:string)
            n1785 = VISA Write(VISA resource name=w2606, write buffer=w2604) -> ()  [unwired: 1 in, 3 out]
          }
          frame #1 {
            "Flushing P3" <- TRUE ("Flushing P3")
          }
        }
      }
      event "Flush Pump 1": Value Change {
        n1786 = event-data() -> ()  [unwired: 7 out]
        n1787 = flat-sequence {
          tunnel: [w2626] -> w2616
          tunnel: w2615 -> [w2619]
          tunnel: w2616 -> [_]
          frame #0 {
            # "set paramaters (rate, volume) for flush, clear volume"
            n1788 = local write "Inject Pump 1"(TRUE ("Inject Pump 1")) -> ()
            n1789 = Number To Decimal String(number="Flush rate (uL/m) P1") -> (decimal integer string=w2642:string)  [unwired: 1 in]
            n1790 = Concatenate Strings("irate  " ("string"), w2642, " u/m" ("string"), "\r") -> (w2644:string)
            n1791 = VISA Write(VISA resource name=w2619, write buffer=w2644) -> (VISA resource name out=w2640:refnum<visa-resource-name>)  [unwired: 1 in, 2 out]
            n1792 = Reciprocal(x="Flush rate (uL/m) P1") -> (1/x=w2623:dbl)
            n1793 = Number To Decimal String(number="Volume (uL) P1") -> (decimal integer string=w2631:string)  [unwired: 1 in]
            n1794 = Multiply(x="Volume (uL) P1", y=w2623) -> (x*y=w2622:dbl)
            n1795 = Concatenate Strings("tvolume  " ("string"), w2631, " u" ("string"), "\r") -> (w2629:string)
            n1796 = Multiply(x=w2622, y=60.0) -> (x*y=→"HP1 Flush Time (s)":dbl)
            n1797 = VISA Write(VISA resource name=w2640, write buffer=w2629) -> (VISA resource name out=w2628:refnum<visa-resource-name>)  [unwired: 1 in, 2 out]
            n1798 = Concatenate Strings("cvolume" ("string"), "\r") -> (w2627:string)
            n1799 = VISA Write(VISA resource name=w2628, write buffer=w2627) -> (VISA resource name out=w2638:refnum<visa-resource-name>)  [unwired: 1 in, 2 out]
            n1800 = Concatenate Strings("irun" ("string"), "\r") -> (w2636:string)
            n1801 = VISA Write(VISA resource name=w2638, write buffer=w2636) -> (VISA resource name out=w2626:refnum<visa-resource-name>)  [unwired: 1 in, 2 out]
          }
          frame #1 {
            "Flushing P1" <- TRUE ("Flushing P3")
          }
        }
      }
      event "Clear Volume": Value Change {
        n1802 = event-data() -> ()  [unwired: 7 out]
        n1803 = Concatenate Strings("cvolume" ("string"), "\r") -> (w2648:string)
        n1804 = VISA Write(VISA resource name=w2647, write buffer=w2648) -> ()  [unwired: 1 in, 3 out]
      }
      event "Clear Volume P3": Value Change {
        n1805 = event-data() -> ()  [unwired: 7 out]
        n1806 = Concatenate Strings("cvolume" ("string"), "\r") -> (w2654:string)
        n1807 = VISA Write(VISA resource name=w2653, write buffer=w2654) -> ()  [unwired: 1 in, 3 out]
        n1808 = local write "Clear Volume P3"(FALSE ("Clear Volume P3")) -> ()
      }
      event "Clear Volume P1": Value Change {
        n1809 = event-data() -> ()  [unwired: 7 out]
        n1810 = Concatenate Strings("cvolume" ("string"), "\r") -> (w2659:string)
        n1811 = local write "Clear Volume P1"(FALSE ("Clear Volume P1")) -> ()
        n1812 = VISA Write(VISA resource name=w2658, write buffer=w2659) -> ()  [unwired: 1 in, 3 out]
      }
      event "Display On P3": Value Change {
        n1813 = event-data() -> ()  [unwired: 7 out]
        n1814 = Select(t="dim 100", s="Display On P3", f="dim 0") -> (s? t:f=w2665:string)
        n1815 = Concatenate Strings(w2665, "\r") -> (w2667:string)
        n1816 = VISA Write(VISA resource name=w2662, write buffer=w2667) -> ()  [unwired: 1 in, 3 out]
      }
      event "Display On P1": Value Change {
        n1817 = event-data() -> ()  [unwired: 7 out]
        n1818 = Select(t="dim 100", s="Display On P1", f="dim 0") -> (s? t:f=w2672:string)
        n1819 = Concatenate Strings(w2672, "\r") -> (w2674:string)
        n1820 = VISA Write(VISA resource name=w2669, write buffer=w2674) -> ()  [unwired: 1 in, 3 out]
      }
      event "Retract Pump 3": Value Change {
        n1821 = event-data() -> ()  [unwired: 7 out]
        n1822 = local write "Retract Pump 3"(FALSE ("Retract Pump 3")) -> ()
        n1823 = case shown="True" "Retract Pump 3" {
          tunnel: w2676 -> [_ w2679]
          frame False {
          }
          frame True {
            n1824 = Number To Decimal String(number="Retract Rate (uL/m)") -> (decimal integer string=w2697:string)  [unwired: 1 in]
            n1825 = Concatenate Strings("wrate  " ("string"), w2697, " u/m" ("string"), "\r") -> (w2699:string)
            n1826 = VISA Write(VISA resource name=w2679, write buffer=w2699) -> (VISA resource name out=w2690:refnum<visa-resource-name>)  [unwired: 1 in, 2 out]
            n1827 = Number To Decimal String(number="Retract Vol 3 (uL)") -> (decimal integer string=w2692:string)  [unwired: 1 in]
            n1828 = Concatenate Strings("tvolume  " ("string"), w2692, " u" ("string"), "\r") -> (w2689:string)
            n1829 = VISA Write(VISA resource name=w2690, write buffer=w2689) -> (VISA resource name out=w2685:refnum<visa-resource-name>)  [unwired: 1 in, 2 out]
            n1830 = Concatenate Strings("cvolume" ("string"), "\r") -> (w2686:string)
            n1831 = VISA Write(VISA resource name=w2685, write buffer=w2686) -> (VISA resource name out=w2680:refnum<visa-resource-name>)  [unwired: 1 in, 2 out]
            n1832 = Concatenate Strings("wrun" ("string"), "\r") -> (w2681:string)
            n1833 = VISA Write(VISA resource name=w2680, write buffer=w2681) -> ()  [unwired: 1 in, 3 out]
          }
        }
      }
      event "Retract Pump 1": Value Change {
        n1834 = event-data() -> ()  [unwired: 7 out]
        n1835 = local write "Retract Pump 1"(FALSE ("Retract Pump 1")) -> ()
        n1836 = case shown="True" "Retract Pump 1" {
          tunnel: w2701 -> [_ w2706]
          frame False {
          }
          frame True {
            n1837 = local read "Retract Rate (uL/m)"() -> (w2704:dbl)
            n1838 = Number To Decimal String(number=w2704) -> (decimal integer string=w2722:string)  [unwired: 1 in]
            n1839 = Concatenate Strings("wrate  " ("string"), w2722, " u/m" ("string"), "\r") -> (w2724:string)
            n1840 = VISA Write(VISA resource name=w2706, write buffer=w2724) -> (VISA resource name out=w2716:refnum<visa-resource-name>)  [unwired: 1 in, 2 out]
            n1841 = Number To Decimal String(number="Retract Vol 1 (uL)") -> (decimal integer string=w2718:string)  [unwired: 1 in]
            n1842 = Concatenate Strings("tvolume  " ("string"), w2718, " u" ("string"), "\r") -> (w2715:string)
            n1843 = VISA Write(VISA resource name=w2716, write buffer=w2715) -> (VISA resource name out=w2712:refnum<visa-resource-name>)  [unwired: 1 in, 2 out]
            n1844 = Concatenate Strings("cvolume" ("string"), "\r") -> (w2713:string)
            n1845 = VISA Write(VISA resource name=w2712, write buffer=w2713) -> (VISA resource name out=w2707:refnum<visa-resource-name>)  [unwired: 1 in, 2 out]
            n1846 = Concatenate Strings("wrun" ("string"), "\r") -> (w2708:string)
            n1847 = VISA Write(VISA resource name=w2707, write buffer=w2708) -> ()  [unwired: 1 in, 3 out]
          }
        }
      }
      event "Flip Green Filter": Value Change {
        n1848 = event-data() -> ()  [unwired: 7 out]
        n1849 = Not(x="Flip Green Filter") -> (.not. x?=w2726:bool)
        n1850 = local write "Flip Green Filter"(w2726) -> ()
        n1851 = flat-sequence {
          tunnel: w2734 -> [w2739]
